vi "Get BLISS_Path to Image Folder.vi"(7 "BLISS Type":enum16{"Reject Images", "PBQA Images"}(ring), 8 "error in (no error)":errorcluster, 11 "Data Parameters in":T1={"Start Time"=timestamp(3690155740.033191 s since 1904-01-01), "Save to Folder"=path "", "Forces in Theater"=[{"Force Commander"="BlissUT124", "Units"=[]}, {"Force Commander"="BlissMP146", "Units"=[]}, {"Force Commander"="BlissMP145", "Units"=[]}, {"Force Commander"="BlissMP140", "Units"=[]}, {"Force Commander"="BlissMP137", "Units"=[]}, {"Force Commander"="BlissMP135", "Units"=[]}, {"Force Commander"="BlissMP134", "Units"=[]}, {"Force Commander"="BlissMP132", "Units"=[]}, {"Force Commander"="BlissMA109", "Units"=[]}, {"Force Commander"="BlissMA107", "Units"=[]}, {"Force Commander"="BlissMA106", "Units"=[]}, {"Force Commander"="BlissMA101", "Units"=[]}, {"Force Commander"="BlissLU118", "Units"=[]}, {"Force Commander"="BlissLU117", "Units"=[]}, {"Force Commander"="BlissLU116", "Units"=[]}, {"Force Commander"="BlissLU115", "Units"=[]}, {"Force Commander"="BlissLU114", "Units"=[]}, {"Force Commander"="BlissLU113", "Units"=[]}, {"Force Commander"="BlissLU111", "Units"=[]}, {"Force Commander"="BlissLL185", "Units"=[]}, {"Force Commander"="BlissLL183", "Units"=[]}, {"Force Commander"="BlissLL173", "Units"=[]}, {"Force Commander"="BlissLL172", "Units"=[]}, {"Force Commander"="BlissLL171", "Units"=[]}, {"Force Commander"="BlissJH103", "Units"=[]}, {"Force Commander"="BlissJH102", "Units"=[]}, {"Force Commander"="BlissJH101", "Units"=[]}, {"Force Commander"="BlissJE116", "Units"=[]}, {"Force Commander"="BlissJE115", "Units"=[]}, {"Force Commander"="BlissJE114", "Units"=[]}, {"Force Commander"="BlissJE111", "Units"=[]}, {"Force Commander"="BlissHD183", "Units"=[]}, {"Force Commander"="BlissHD182", "Units"=[]}, {"Force Commander"="BlissHD181", "Units"=[]}, {"Force Commander"="BlissGPDFFPL", "Units"=[]}, {"Force Commander"="BlissEUWIPES", "Units"=[]}, {"Force Commander"="BlissEU179", "Units"=[]}, {"Force Commander"="BlissEU178", "Units"=[]}, {"Force Commander"="BlissEU177", "Units"=[]}, {"Force Commander"="Blissdvds02", "Units"=[]}, {"Force Commander"="BlissDOWIPES", "Units"=[]}, {"Force Commander"="BlissCR022", "Units"=[]}, {"Force Commander"="BlissCR021", "Units"=[]}, {"Force Commander"="BlissCG167", "Units"=[]}, {"Force Commander"="BlissCG166", "Units"=[]}, {"Force Commander"="BlissCG161", "Units"=[]}, {"Force Commander"="BlissCG160", "Units"=[]}, {"Force Commander"="BlissCG159", "Units"=[]}, {"Force Commander"="BlissCG158", "Units"=[]}, {"Force Commander"="BlissCG157", "Units"=[]}, {"Force Commander"="BlissCG156", "Units"=[]}, {"Force Commander"="BlissCG151", "Units"=[]}, {"Force Commander"="BlissCB172", "Units"=[]}, {"Force Commander"="BlissCB171", "Units"=[]}, {"Force Commander"="BlissCB108", "Units"=[]}, {"Force Commander"="BlissCB107", "Units"=[]}, {"Force Commander"="BlissBV181", "Units"=[]}, {"Force Commander"="BlissBV162", "Units"=[]}, {"Force Commander"="BlissAK177", "Units"=[]}, {"Force Commander"="BlissAK176", "Units"=[]}, {"Force Commander"="BlissAK175", "Units"=[]}, {"Force Commander"="BlissAK174", "Units"=[]}, {"Force Commander"="BlissAK173", "Units"=[]}, {"Force Commander"="BlissAK172", "Units"=[]}, {"Force Commander"="BlissAK171", "Units"=[]}, {"Force Commander"="BlissAK139", "Units"=[]}, {"Force Commander"="BlissAK134", "Units"=[]}, {"Force Commander"="BlissAK131", "Units"=[]}, {"Force Commander"="BlissAH163", "Units"=[]}, {"Force Commander"="BlissAH162", "Units"=[]}, {"Force Commander"="BlissAH161", "Units"=[]}, {"Force Commander"="BlissAH122", "Units"=[]}, {"Force Commander"="BlissAH121", "Units"=[]}, {"Force Commander"="BlissAD106", "Units"=[]}, {"Force Commander"="BlissAD104", "Units"=[]}, {"Force Commander"="BlissAB105", "Units"=[]}, {"Force Commander"="BlissAB104", "Units"=[]}]}) -> (0 "error out":errorcluster, 2 "Dates (folders)":string[](array[string]), 3 "Server Images Path":path, 4 "Server Name":string)   [LabVIEW 2020]
uses:
  MC5e Squad_Info.ctl
  MC5e Unit_Status_List.ctl
  MC5e Data_Parameters.ctl
  MC5e Terrain types.ctl
  Location.ctl
  MC5e Unit.ctl
  MC5e Force.ctl
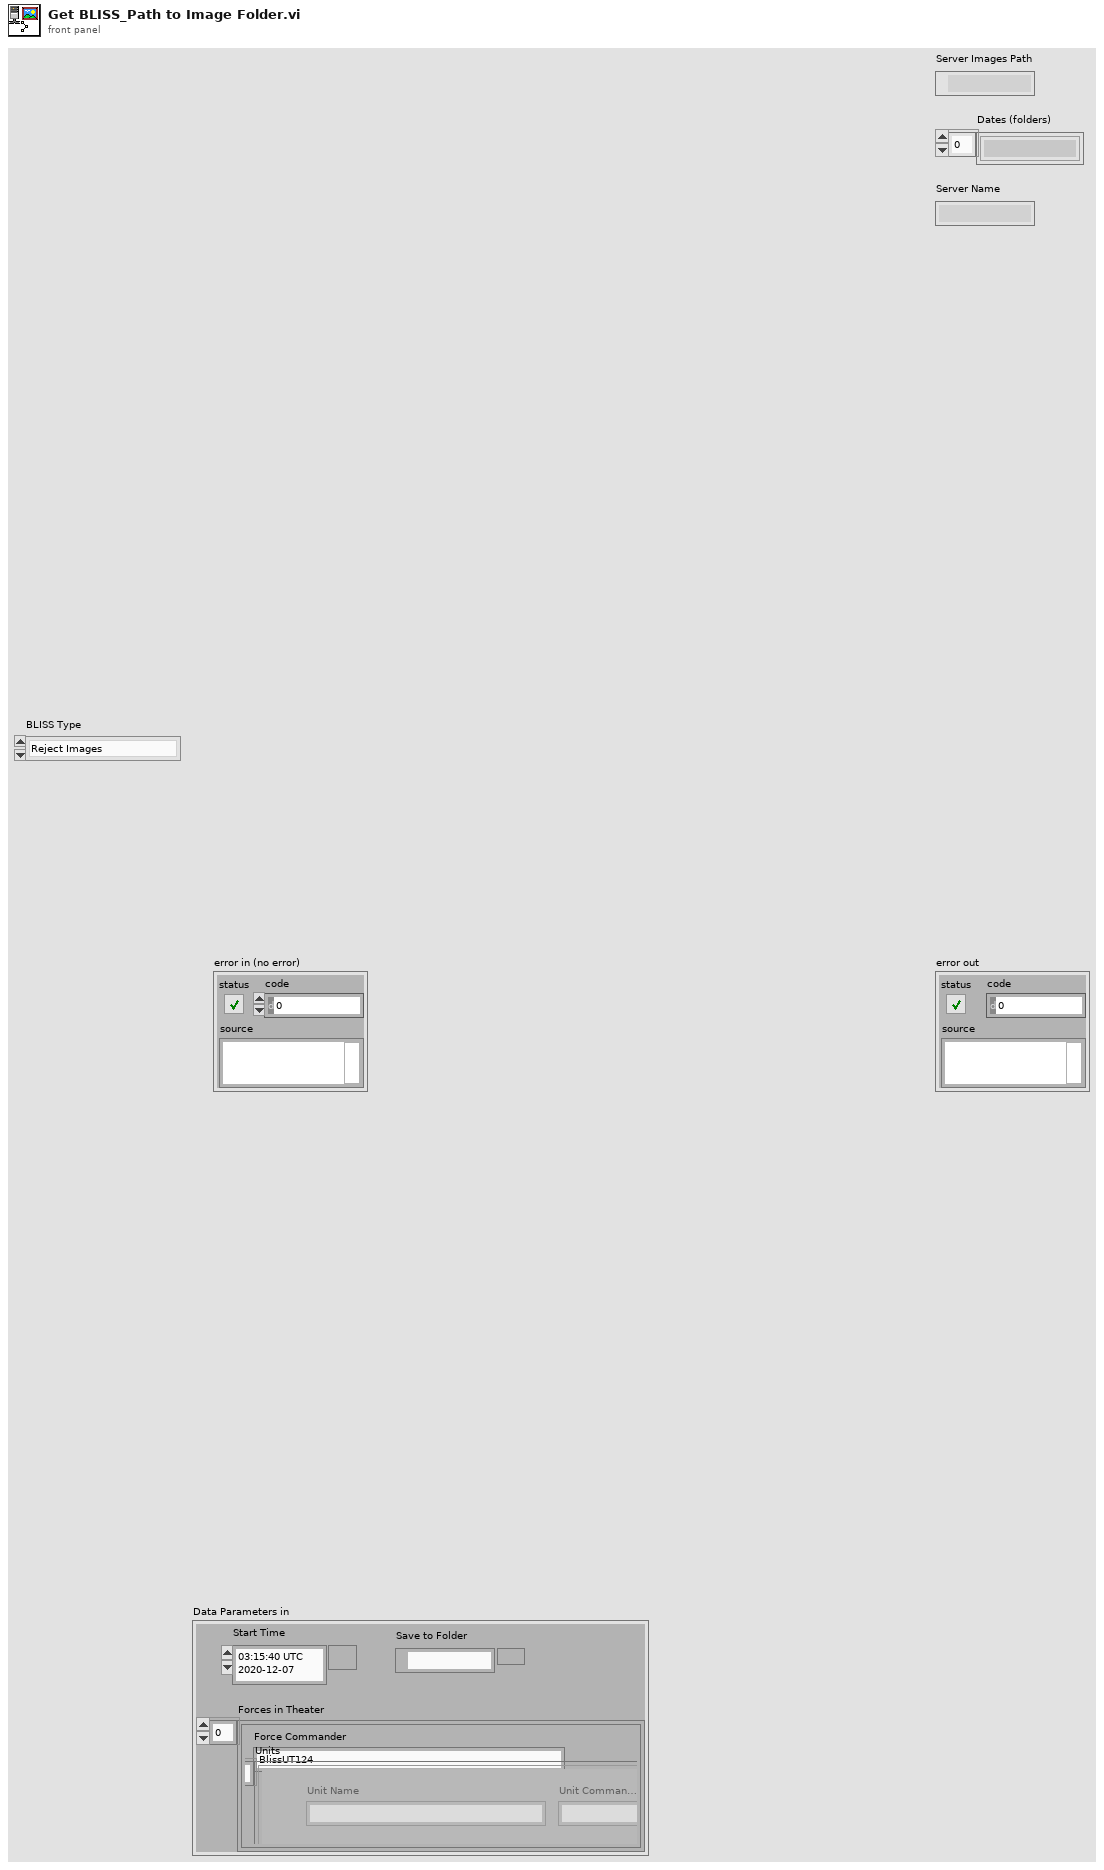
[diagram p1: front panel]
types:
  T1 = typedef "MC5e Data_Parameters.ctl" = cluster{"Start Time":timestamp, "Save to Folder":path, "Forces in Theater":T2[]}
  T2 = typedef "MC5e Force.ctl" = cluster{"Force Commander":string, "Units":T3[]}
  T3 = typedef "MC5e Unit.ctl" = cluster{"Squad List":T4, "Unit Fatigue Level":enum16{"Not Fatigued", "Fatigued", "Seriously Fatigued"}, "Flying Unit":bool, "Mounted Unit":bool, "Difficult Terrain Types":T6, "Full BR":dbl, "Defending from Stronghold":bool, "Speed":dbl, "Capacity %":dbl, "Morale":dbl, "Current BR":dbl, "Location":T7, "Unit Name":string, "Unit Commander":string, "Unit Notes":string}
  T4 = typedef "MC5e Unit_Status_List.ctl" = T5[]
  T5 = typedef "MC5e Squad_Info.ctl" = cluster{"Squad Name":string, "# Soldiers":dbl, "Battle Rating":dbl, "Flying":bool, "Mounted":bool, "Speed":dbl, "Range":dbl, "Morale":dbl, "Token Image":variant, "Max Endurance":dbl, "Current Endurance":dbl, "Difficult Terrain":T6}
  T6 = typedef "MC5e Terrain types.ctl" = cluster{"Artic / snow / ice)":bool, "Coast":bool, "Desert / sand":bool, "Forest / woodland":bool, "Grassland / plains":bool, "Mountain / canyons":bool, "Underdark / caverns":bool, "Acquatic / rivers, lakes, ocean":bool}
  T7 = typedef "Location.ctl" = cluster{"X coordinate":dbl, "Y coordinate":dbl}
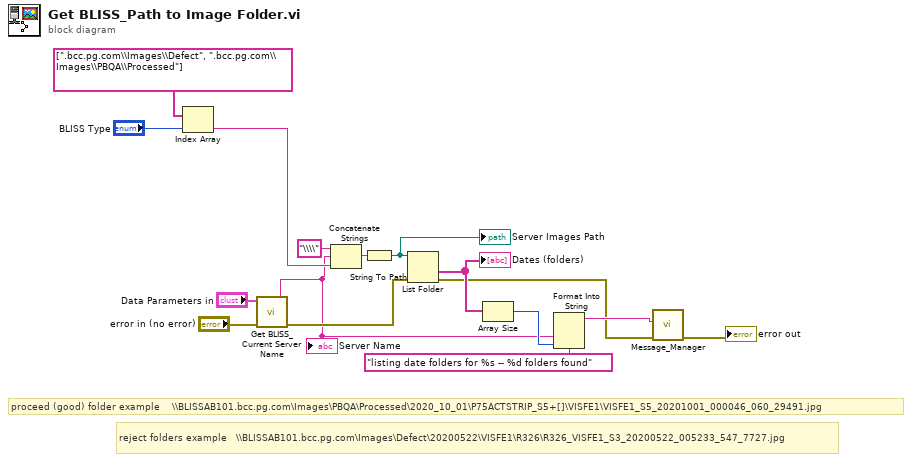
[diagram p0: block diagram]
diagram:
  # "reject folders example   \\\\BLISSAB101.bcc.pg.com\\Images\\Defect\\20200522\\VISFE1\\R326\\R326_VISFE1_S3_20200522_005233_547_7727.jpg"
  # "proceed (good) folder example    \\\\BLISSAB101.bcc.pg.com\\Images\\PBQA\\Processed\\2020_10_01\\P75ACTSTRIP_S5+[]\\VISFE1\\VISFE1_S5_20201001_000046_060_29491.jpg"
  n1 = Index Array(array=string[] [".bcc.pg.com\\Images\\Defect", ".bcc.pg.com\\Images\\PBQA\\Processed"], index="BLISS Type") -> (element=w9:string)
  n2 = call "Get BLISS_Current Server Name.vi"("error in"="error in (no error)", "Data Parameters in"="Data Parameters in") -> ("error out"=w15:errorcluster, "Server Name"=w2:string)  [unwired: 6 in, 2 out]
  "Server Name" <- w2
  n3 = Concatenate Strings("\\\\" ("string"), w2, w9) -> (w13:string)
  n4 = String To Path(string=w13) -> (path=w12:path)
  "Server Images Path" <- w12
  n5 = List Folder(path=w12, error in=w15) -> (folder names=w6:string[], error out=w4:errorcluster)  [unwired: 2 in, 2 out]
  "Dates (folders)" <- w6
  n6 = Array Size(array=w6) -> (size(s)=w5:i32)
  n7 = Format Into String(format string="listing date folders for %s -- %d folders found", w2, w5) -> (resulting string=w7:string)  [unwired: 2 in, 1 out]
  n8 = call "Message_Manager.vi"("error in"=w4, "New Entry"=w7) -> ("error out"=→"error out":errorcluster)  [unwired: 4 in, 5 out]
